vi "Main.vi"(10 "DAQ Type":enum16{"Hardware", "Simulation"}(ring), 11 "Module Admin":refnum<class "Delacor_lib_QMH_Module Admin.lvclass">) -> ()   [LabVIEW 2021, in "Func Generator.lvlib"]
doc: "This template is based off of the Queued Message Handler design pattern and the Queued Message Handler project template that ships with LabVIEW.\n\nThe main difference is that the queue is private to this module and communication between modules is performed via Broadcast and Request events.\n\nRequest events are wrapped in public API methods and are handled in the Event Handling Loop (EHL) of this VI. Any module can register for Broadcast events sent by this module. The EHL generates messages based on user interface actions.\n\nThe Message Handling Loop (MHL) processes messages generated by the EHL, or by other messages. The messages are string values, so new messages can be added easily to the Message Cases case structure in the MHL. Each message cluster can also provide an optional value for Message Data, which is a variant that can be converted to whatever message-specific data is required.\n_____\nBased on DQMH Project Template 6.1.0.94."
uses:
  Func Generator.lvlib
  <vilib>/Delacor/Delacor QMH/Libraries/Module Admin_class/Delacor_lib_QMH_Module Admin.lvclass
  Class/Agilent 33210A/Agilent 33210A.lvclass
  C:/repository/common_ATE/Libraries/Func Generator/Class/Abstract/Abstract.lvclass
  Class/Abstract/Abstract.lvclass
  Module Data--cluster.ctl
  Instrument Setting.ctl
  <vilib>/Delacor/Delacor QMH/Libraries/Message Queue_class/Delacor_lib_QMH_Message Queue.lvclass/Delacor_lib_QMH_Message Queue.ctl
  Stop Argument--cluster.ctl
  <vilib>/Delacor/Delacor QMH/Libraries/Module Admin_class/Delacor_lib_QMH_Module Admin.lvclass/Delacor_lib_QMH_Module Admin.ctl
  REQ Initialize Hardware Argument--cluster.ctl
  REQ Initialize Hardware (Reply Payload)--cluster.ctl
  REQ Enable Output Argument--cluster.ctl
  REQ Set Output Impedance Argument--cluster.ctl
  REQ Config Std Waveform Argument--cluster.ctl
  REQ Config Freq Sweep Argument--cluster.ctl
  REQ Self Test Argument--cluster.ctl
  REQ Close Ref Argument--cluster.ctl
  <vilib>/Utility/miscctls.llb/LVPointTypeDef.ctl
  <vilib>/Delacor/Delacor QMH/Libraries/Message Queue_class/Delacor_lib_QMH_Enqueue Message (Single).vi
  <vilib>/Delacor/Delacor QMH/Libraries/Module Admin_class/Delacor_lib_QMH_Get External Launch.vi
  <vilib>/Utility/error.llb/Error Cluster From Error Code.vi
  <vilib>/ErrorRing/Error Ring.xnode
  <vilib>/Delacor/Delacor QMH/Libraries/Message Queue_class/Delacor_lib_QMH_Message Queue.lvclass
panel:
  out "error out":errorcluster
  out "Status":string
  in  "Simulate MHL Error":bool
  in  "Simulate EHL Error":bool
  # "Other QMH Modules communicate with this Module via its Public API (wrappers for its Request Events).\n\nThis Module communicates with other Modules via its Broadcast Events.\nAny module that wants to get these messages, just registers for this module's Broadcast events."
  # "This template is for the Delacor Modified Queued Message Handler design pattern.\n\nSee the block diagram for more information on how to use this template."
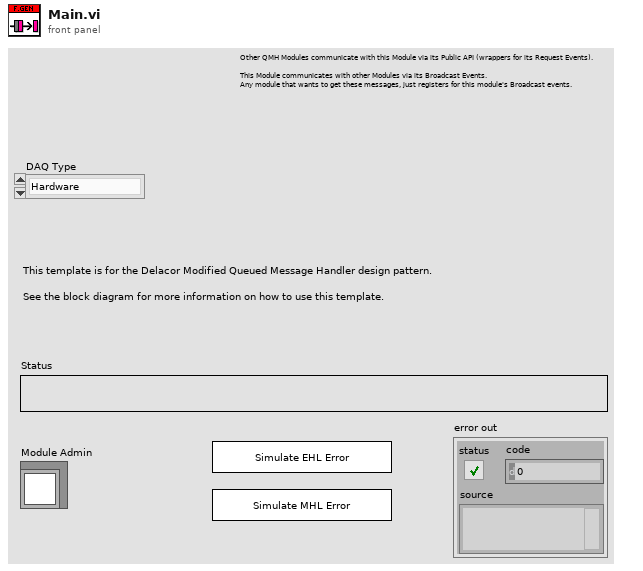
[diagram p1: front panel]
types:
  T1 = typedef "Func Generator.lvlib/Request Events--cluster.ctl" = cluster{"Stop Module":refnum<user-event>, "Show Panel":refnum<user-event>, "Hide Panel":refnum<user-event>, "Get Module Execution Status":refnum<user-event>, "Show Diagram":refnum<user-event>, "REQ Initialize Hardware":refnum<user-event>, "REQ Enable Output":refnum<user-event>, "REQ Set Output Impedance":refnum<user-event>, "REQ Config Std Waveform":refnum<user-event>, "REQ Config Freq Sweep":refnum<user-event>, "REQ Self Test":refnum<user-event>, "REQ Close Ref":refnum<user-event>}
  T2 = typedef "Func Generator.lvlib/Module Data--cluster.ctl" = cluster{"Status":string, "Abstract.lvclass":refnum<class "Abstract.lvclass">, "Connection Setting":T3}
  T3 = typedef "Func Generator.lvlib/Instrument Setting.ctl" = cluster{"Connection Ref":variant, "Serial Configuration":cluster{"Baud Rate":u32, "Parity":u16, "Data Bits":u16, "Flow Control":u16}}
  T4 = enum32{"invalid lock state", "Not Locked", "Locked (No Password)", "Password-protected"}
  T5 = typedef "Func Generator.lvlib/Stop Argument--cluster.ctl" = cluster{"Origin":string, "Exit via Stop Module Req?":bool, "Wait for Module to stop?":bool}
  T6 = typedef "Func Generator.lvlib/REQ Initialize Hardware Argument--cluster.ctl" = cluster{"Connection Setting":T3, "Wait Notifier":refnum<notifier>, "wait for reply":bool}
  T7 = typedef "Func Generator.lvlib/REQ Enable Output Argument--cluster.ctl" = cluster{"Output":bool}
  T8 = typedef "Func Generator.lvlib/REQ Set Output Impedance Argument--cluster.ctl" = cluster{"User-Defined Impedance (50 Ohms)":dbl, "Impedance (0: 50 Ohms)":u16}
  T9 = typedef "Func Generator.lvlib/REQ Config Std Waveform Argument--cluster.ctl" = cluster{"Std Waveform Setting":cluster{"Waveform Function (1: Sine)":u16, "Frequency (1000 Hz)":dbl, "Amplitude (1)":dbl, "Unit (0: Vpp)":u16, "DC Offset (0.00 V)":dbl}}
  T10 = typedef "Func Generator.lvlib/REQ Config Freq Sweep Argument--cluster.ctl" = cluster{"Freq Sweep Setting":cluster{"Sweep Spacing (0: Linear)":u16, "Sweep Time (1.00 s)":dbl, "Stop  Frequency (1000.0 Hz)":dbl, "Start Frequency (100.0 Hz)":dbl, "Enable/Disable Freq Sweep":bool}}
  T11 = typedef "Func Generator.lvlib/REQ Self Test Argument--cluster.ctl" = cluster{"Boolean":bool}
  T12 = typedef "Func Generator.lvlib/REQ Close Ref Argument--cluster.ctl" = cluster{"Boolean":bool}
  T13 = typedef "LVPointTypeDef.ctl" = cluster{"Horizontal":i16, "Vertical":i16}
  T14 = enum32{"Invalid", "Standard", "Closed", "Hidden", "Minimized", "Maximized"}
  T15 = typedef "Func Generator.lvlib/REQ Initialize Hardware (Reply Payload)--cluster.ctl" = cluster{"Connect?":bool, "error":errorcluster}
  T16 = cluster{"Waveform Function (1: Sine)":u16, "Frequency (1000 Hz)":dbl, "Amplitude (1)":dbl, "Unit (0: Vpp)":u16, "DC Offset (0.00 V)":dbl}
  T17 = cluster{"Sweep Spacing (0: Linear)":u16, "Sweep Time (1.00 s)":dbl, "Stop  Frequency (1000.0 Hz)":dbl, "Start Frequency (100.0 Hz)":dbl, "Enable/Disable Freq Sweep":bool}
  T18 = typedef "Instrument Setting.ctl" = cluster{"Connection Ref":variant, "Serial Configuration":cluster{"Baud Rate":u32, "Parity":u16, "Data Bits":u16, "Flow Control":u16}}
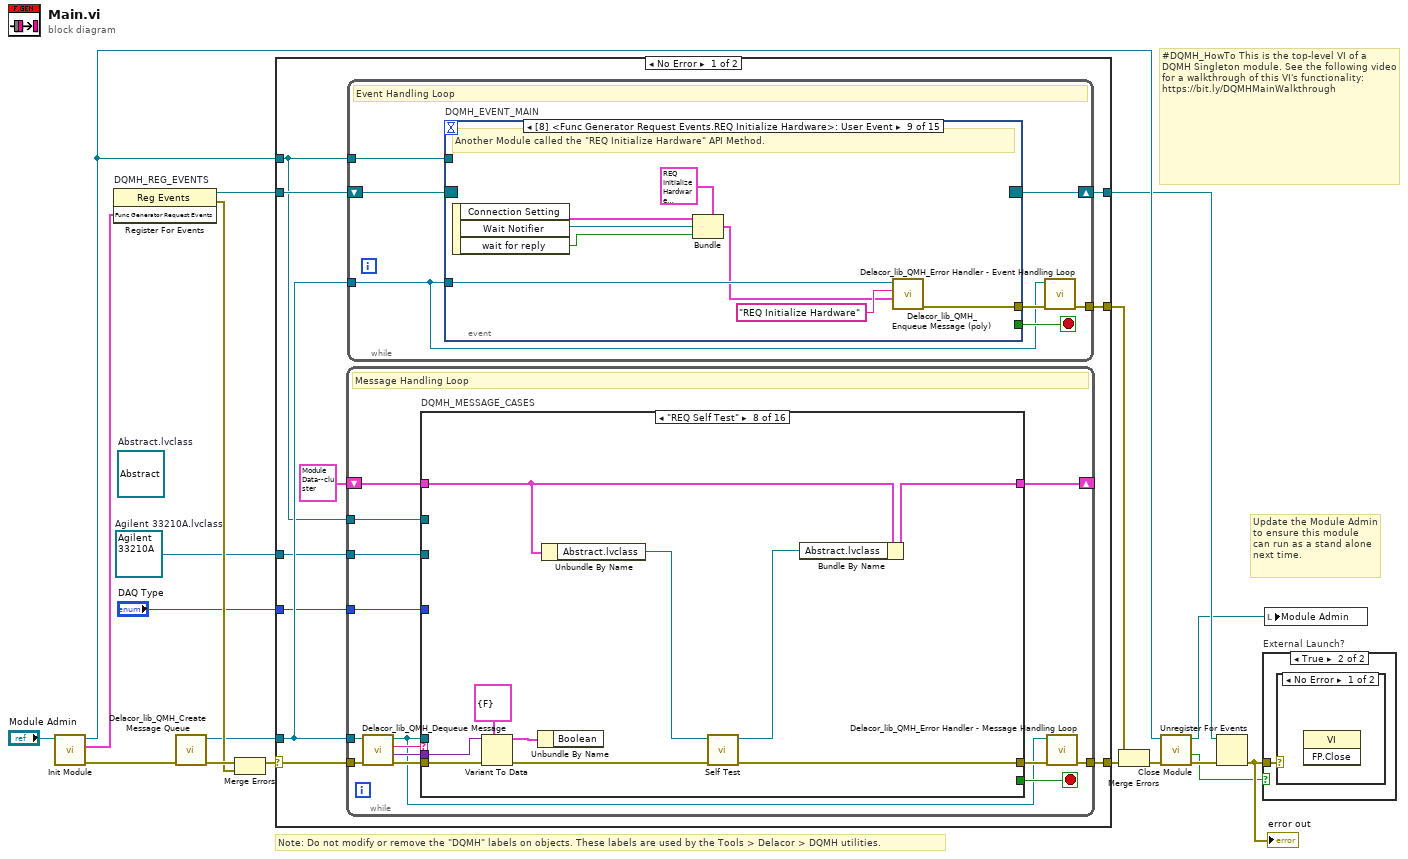
[diagram p0: block diagram]
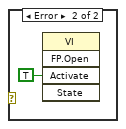
[diagram p3: hidden frame]
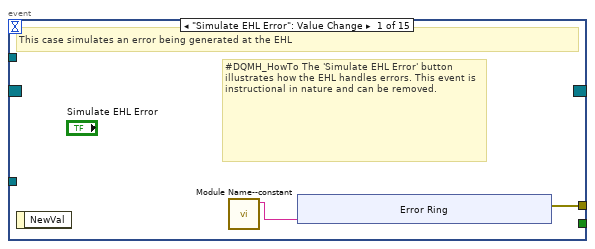
[diagram p4: hidden frame]
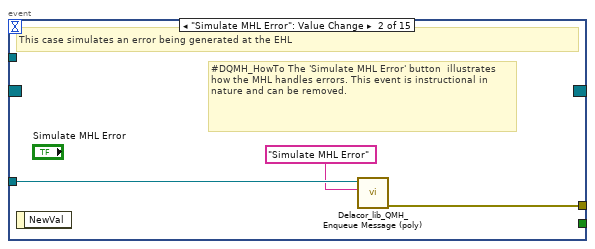
[diagram p5: hidden frame]
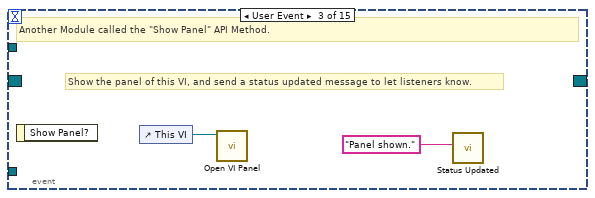
[diagram p6: hidden frame]
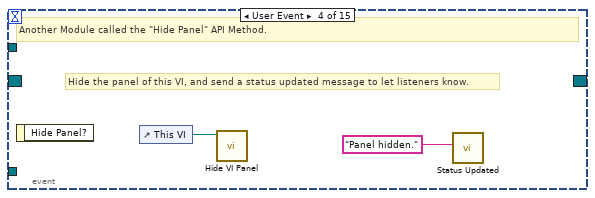
[diagram p7: hidden frame]
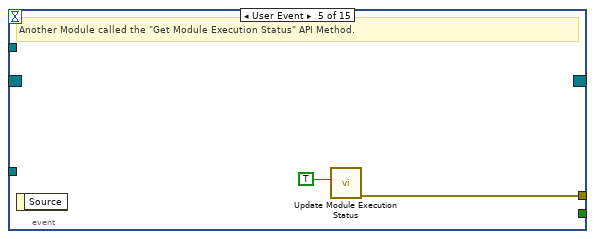
[diagram p8: hidden frame]
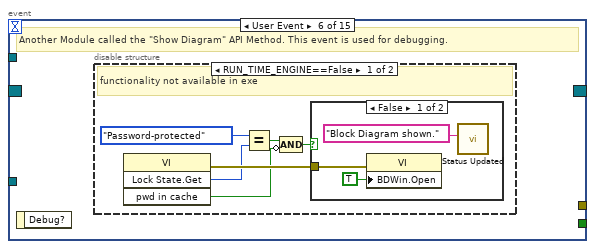
[diagram p9: hidden frame]
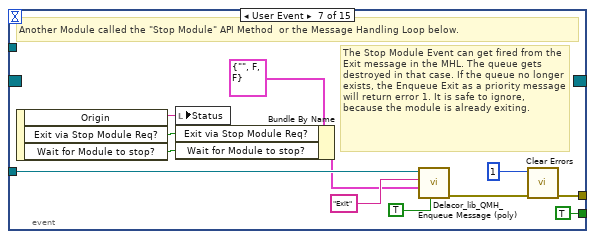
[diagram p12: hidden frame]
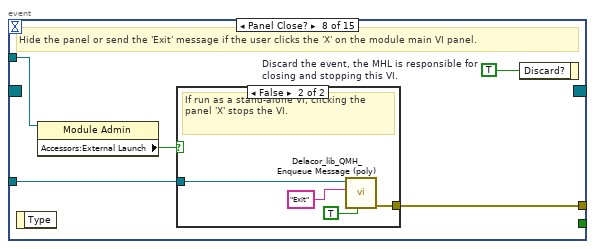
[diagram p13: hidden frame]
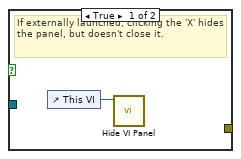
[diagram p14: hidden frame]
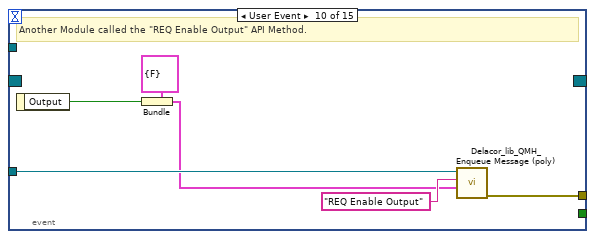
[diagram p15: hidden frame]
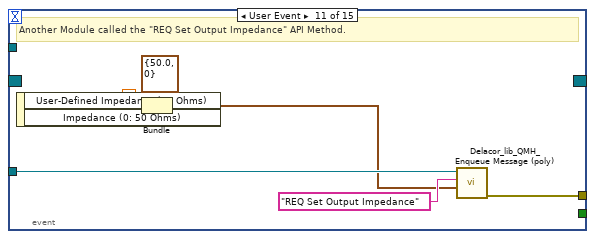
[diagram p16: hidden frame]
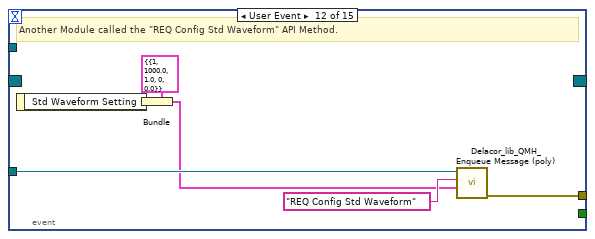
[diagram p17: hidden frame]
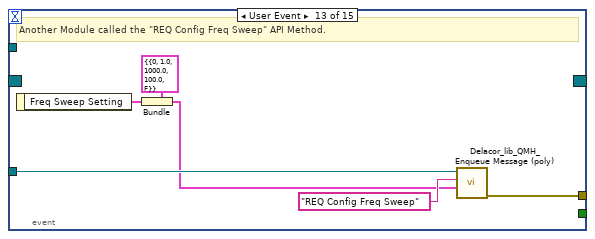
[diagram p18: hidden frame]
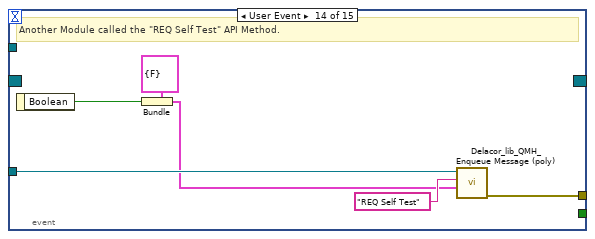
[diagram p19: hidden frame]
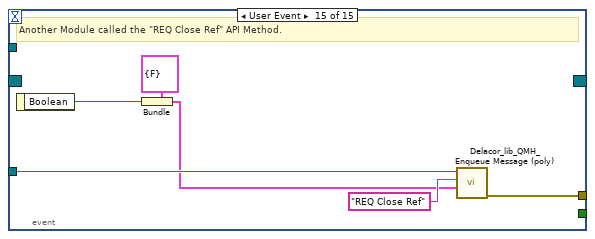
[diagram p20: hidden frame]
diagram:
  w2 = refnum<class "Agilent 33210A.lvclass"> refnum  # Agilent 33210A.lvclass
  (unwired) refnum<class "Abstract.lvclass"> refnum  # Abstract.lvclass
  # "#DQMH_HowTo This is the top-level VI of a DQMH Singleton module. See the following video for a walkthrough of this VI's functionality: https://bit.ly/DQMHMainWalkthrough"
  # "Note: Do not modify or remove the \"DQMH\" labels on objects. These labels are used by the Tools > Delacor > DQMH utilities."
  # "Update the Module Admin to ensure this module can run as a stand alone next time."
  n1 = call "Init Module.vi"("Singleton Module Admin in"="Module Admin") -> ("error out"=w18:errorcluster, "Func Generator Request Events"=w7:T1, "Singleton Module Admin out"=w10:refnum<class "Delacor_lib_QMH_Module Admin.lvclass">)  [unwired: 8 in]
  n2 = register-events "DQMH_REG_EVENTS"(w7) -> (reference out=w8:refnum<event-registration>, error out=w11:errorcluster)  [unwired: 2 in]
  n3 = call <vilib>:"Delacor_lib_QMH_Create Message Queue.vi"("error in"=w18) -> ("error out"=w13:errorcluster, "Message Queue"=w6:refnum<class "Delacor_lib_QMH_Message Queue.lvclass">)  [unwired: 9 in]
  n4 = Merge Errors(w13, w11) -> (w12:errorcluster)
  n5 = case shown="No Error" w12 {
    selector: w12 -> [w27 w331]
    tunnel: [w29 w330] -> w19
    tunnel: [w26 w336] -> w9
    tunnel: w8 -> [w24 w336]
    tunnel: w6 -> [w23 w329]
    tunnel: [w28 _] -> w16
    tunnel: w10 -> [w22 w332]
    tunnel: w2 -> [w21 _]
    tunnel: "DAQ Type" -> [w20 _]
    frame No Error {
      n6 = while {
        tunnel: w23 -> [w135]
        shift-right: [w139] -> _
        shift-left: T2 {"Status"="", "Abstract.lvclass"=refnum, "Connection Setting"={"Connection Ref"=variant, "Serial Configuration"={"Baud Rate"=9600, "Parity"=0, "Data Bits"=8, "Flow Control"=4}}} ("Data Cluster") -> [w140]
        tunnel: w27 -> [w143]
        tunnel: [w141] -> w29
        tunnel: w22 -> [w133]
        tunnel: w21 -> [w132]
        tunnel: w20 -> [w131]
        stop <- w138 stop-if-true
        # "Message Handling Loop"
        n7 = call-dynamic "Delacor_lib_QMH_Dequeue Message.vi"("error in"=w143, "Message Queue in"=w135) -> ("error out"=w142:errorcluster, "Message Data"=w136:variant, "Message"=w137:string, "Message Queue out"=w134:refnum<class "Delacor_lib_QMH_Message Queue.lvclass">)  [unwired: 6 in]
        n8 = case "DQMH_MESSAGE_CASES" shown="\"REQ Self Test\"" w137 {
          selector: w137 -> [_ _ _ _ _ _ _ _ _ _ _ _ _ _ _ w316]
          tunnel: w134 -> [_ _ _ _ _ _ _ _ w248 _ _ _ _ w281 w309 _]
          tunnel: w142 -> [w163 w167 w185 w198 w210 w221 w232 w242 w250 w261 w264 w266 w271 w288 w314 w318]
          tunnel: [w161 w167 w173 w188 w199 w212 w222 w233 w249 w252 w263 w266 w270 w284 w311 w319] -> w144
          tunnel: w140 -> [w152 w166 w169 w192 w205 w216 w226 w237 w246 w256 w262 w265 w268 w283 w299 w317]
          tunnel: [w151 w166 w175 w190 w201 w214 w224 w235 w246 w254 w262 w265 w268 w283 w297 w317] -> w139
          tunnel: [_ _ _ _ _ _ _ _ _ _ _ _ _ _ w308 _] -> w138
          tunnel: w136 -> [_ _ w184 w197 w209 w220 w231 w241 _ w260 _ _ _ w282 w307 _]
          tunnel: w133 -> [w153 _ _ _ _ _ _ _ _ _ _ _ _ w280 w302 _]
          tunnel: w132 -> [w145 _ _ _ _ _ _ _ _ _ _ _ _ _ _ _]
          tunnel: w131 -> [_ _ w176 _ _ _ _ _ _ _ _ _ _ _ _ _]
          frame "Initialize" {
            w147 = "Initial Message" ("Initial Message")
            # "Initialize - Any operation that needs to be done before the module can receive messages. Synchronize Caller Events.vi will inform Start Module.vi that the module has launched and is ready to receive messages. Module Did Init.vi will broadcast that the module initialized."
            n9 = call "Synchronize Caller Events.vi"("error in (no error)"=w163, "Singleton Module Admin in"=w153) -> ("error out"=w162:errorcluster, "Singleton Module Admin out"=w148:refnum<class "Delacor_lib_QMH_Module Admin.lvclass">)  [unwired: 8 in]
            n10 = property class="Module Admin"(reference=w148) -> ("Accessors:External Launch"=w157:bool)  [unwired: 1 in, 2 out]
            n11 = Select(t=T14."Hidden" ("State"), s=w157, f=T14."Standard" ("State")) -> (s? t:f=w154:T14)
            n12 = call "Module Name--constant.vi"() -> ("Module Name"=w160:string)  [unwired: 11 in]
            n13 = property class="VI"("Front Panel.Title"=w160) -> (reference out=w159:refnum<vi>, error out=w165:errorcluster)  [unwired: 2 in]
            n14 = call "Module Name--constant.vi"() -> ("Module Name"=w149:string)  [unwired: 11 in]
            n15 = Bundle By Name(cluster=w152, "Status"=w147, "Abstract.lvclass"=w145) -> (w151:T2)
            n16 = invoke class="VI" method="FP.Open"(reference=w159, error in=w165, "State"=w154) -> (reference out=w158:refnum<vi>, error out=w164:errorcluster)  [unwired: 2 in, 3 out]
            n17 = call "Module Did Init.vi"("error in (no error)"=w162, "Initialized?"=TRUE, "Origin"=w149) -> ("error out"=w161:errorcluster)  [unwired: 8 in]
            n18 = invoke class="VI" method="FP.Center"(reference=w158, error in=w164) -> ()  [unwired: 1 in, 3 out]
            n19 = property on="Pane" class="Pane"("Origin"=T13 {"Horizontal"=0, "Vertical"=0}) -> ()  [unwired: 2 in, 2 out]
            "Status" <- w147
          }
          frame "---Module Specific---" {
            # "Separator -- The following cases handle messages specific to this Module."
          }
          frame "REQ Initialize Hardware" {
            n20 = Variant To Data(error in=w185, type=T6 {"Connection Setting"={"Connection Ref"=variant, "Serial Configuration"={"Baud Rate"=9600, "Parity"=0, "Data Bits"=8, "Flow Control"=4}}, "Wait Notifier"=refnum, "wait for reply"=FALSE} ("REQ Initialize Hardware Argument"), Variant=w184) -> (data=w182:T6, error out=w177:errorcluster)
            n21 = Unbundle By Name(w182) -> ("Wait Notifier"=w181:refnum<notifier>, "wait for reply"=w180:bool, "Connection Setting"=w170:T3)
            n22 = Unbundle By Name(w169) -> ("Abstract.lvclass"=w168:refnum<class "Abstract.lvclass">)
            n23 = call-dynamic "Initialize Hardware.vi"("error in (no error)"=w177, "DAQ Type"=w176, "Connection Setting"=w170, "Abstract in"=w168) -> ("error out"=w173:errorcluster, "Abstract out"=w174:refnum<class "Abstract.lvclass">)  [unwired: 6 in]
            n24 = Bundle By Name(cluster=w169, "Connection Setting"=w170, "Abstract.lvclass"=w174) -> (w175:T2)
            n25 = Unbundle By Name(w173) -> ("status"=w172:bool)
            n26 = Not(x=w172) -> (.not. x?=w171:bool)
            n27 = Bundle By Name(cluster=T15 {"Connect?"=FALSE, "error"={"status"=FALSE, "code"=0, "source"=""}} ("REQ Initialize Hardware (Reply Payload)"), "Connect?"=w171) -> (w179:T15)
            n28 = case shown="True" w180 {
              tunnel: w181 -> [_ w187]
              tunnel: w179 -> [_ w186]
              frame False {
              }
              frame True {
                n29 = Send Notification(notification=w186, notifier=w187) -> ()  [unwired: 1 in, 2 out]
              }
            }
          }
          frame "REQ Enable Output" {
            n30 = Variant To Data(error in=w198, type=T7 {"Output"=FALSE} ("REQ Enable Output Argument"), Variant=w197) -> (data=w195:T7, error out=w194:errorcluster)
            n31 = Unbundle By Name(w195) -> ("Output"=w193:bool)
            n32 = Unbundle By Name(w192) -> ("Abstract.lvclass"=w191:refnum<class "Abstract.lvclass">)
            n33 = call-dynamic "Enable Output.vi"("error in (no error)"=w194, "Output"=w193, "Abstract in"=w191) -> ("error out"=w188:errorcluster, "Abstract out"=w189:refnum<class "Abstract.lvclass">)  [unwired: 7 in]
            n34 = Bundle By Name(cluster=w192, "Abstract.lvclass"=w189) -> (w190:T2)
          }
          frame "REQ Set Output Impedance" {
            n35 = Variant To Data(error in=w210, type=T8 {"User-Defined Impedance (50 Ohms)"=50.0, "Impedance (0: 50 Ohms)"=0} ("REQ Set Output Impedance Argument"), Variant=w209) -> (data=w207:T8, error out=w206:errorcluster)
            n36 = Unbundle By Name(w207) -> ("Impedance (0: 50 Ohms)"=w203:u16, "User-Defined Impedance (50 Ohms)"=w202:dbl)
            n37 = Unbundle By Name(w205) -> ("Abstract.lvclass"=w204:refnum<class "Abstract.lvclass">)
            n38 = call-dynamic "Set Output Impedance.vi"("error in (no error)"=w206, "User-Defined Impedance (50 Ohms)"=w202, "Impedance (0: 50 Ohms)"=w203, "Abstract in"=w204) -> ("error out"=w199:errorcluster, "Abstract out"=w200:refnum<class "Abstract.lvclass">)  [unwired: 6 in]
            n39 = Bundle By Name(cluster=w205, "Abstract.lvclass"=w200) -> (w201:T2)
          }
          frame "REQ Config Std Waveform" {
            n40 = Variant To Data(error in=w221, type=T9 {"Std Waveform Setting"={"Waveform Function (1: Sine)"=1, "Frequency (1000 Hz)"=1000.0, "Amplitude (1)"=1.0, "Unit (0: Vpp)"=0, "DC Offset (0.00 V)"=0.0}} ("REQ Config Std Waveform Argument"), Variant=w220) -> (data=w218:T9, error out=w217:errorcluster)
            n41 = Unbundle By Name(w218) -> ("Std Waveform Setting"=w211:T16)
            n42 = Unbundle By Name(w216) -> ("Abstract.lvclass"=w215:refnum<class "Abstract.lvclass">)
            n43 = call-dynamic "Configure Standard Waveform.vi"("error in (no error)"=w217, "Std Waveform Setting"=w211, "Abstract in"=w215) -> ("error out"=w212:errorcluster, "Abstract out"=w213:refnum<class "Abstract.lvclass">)  [unwired: 7 in]
            n44 = Bundle By Name(cluster=w216, "Abstract.lvclass"=w213) -> (w214:T2)
          }
          frame "REQ Config Freq Sweep" {
            n45 = Variant To Data(error in=w232, type=T10 {"Freq Sweep Setting"={"Sweep Spacing (0: Linear)"=0, "Sweep Time (1.00 s)"=1.0, "Stop  Frequency (1000.0 Hz)"=1000.0, "Start Frequency (100.0 Hz)"=100.0, "Enable/Disable Freq Sweep"=FALSE}} ("REQ Config Freq Sweep Argument"), Variant=w231) -> (data=w229:T10, error out=w228:errorcluster)
            n46 = Unbundle By Name(w229) -> ("Freq Sweep Setting"=w227:T17)
            n47 = Unbundle By Name(w226) -> ("Abstract.lvclass"=w225:refnum<class "Abstract.lvclass">)
            n48 = call-dynamic "Configure Frequency Sweep.vi"("error in (no error)"=w228, "Freq Sweep Setting"=w227, "Abstract in"=w225) -> ("error out"=w222:errorcluster, "Abstract out"=w223:refnum<class "Abstract.lvclass">)  [unwired: 7 in]
            n49 = Bundle By Name(cluster=w226, "Abstract.lvclass"=w223) -> (w224:T2)
          }
          frame "REQ Self Test" {
            n50 = Variant To Data(error in=w242, type=T11 {"Boolean"=FALSE} ("REQ Self Test Argument"), Variant=w241) -> (data=w239:T11, error out=w238:errorcluster)
            n51 = Unbundle By Name(w239) -> ()  [unwired: 1 out]
            n52 = Unbundle By Name(w237) -> ("Abstract.lvclass"=w236:refnum<class "Abstract.lvclass">)
            n53 = call-dynamic "Self Test.vi"("error in (no error)"=w238, "Abstract in"=w236) -> ("error out"=w233:errorcluster, "Abstract out"=w234:refnum<class "Abstract.lvclass">)  [unwired: 8 in]
            n54 = Bundle By Name(cluster=w237, "Abstract.lvclass"=w234) -> (w235:T2)
          }
          frame "REQ Reconnect" {
            # "Duplicate this frame when creating new messages.  Change this comment in the duplicated frame to describe this message."
            n55 = Unbundle By Name(w246) -> ("Connection Setting"=w245:T3)
            n56 = Bundle By Name(cluster=T6 {"Connection Setting"={"Connection Ref"=variant, "Serial Configuration"={"Baud Rate"=9600, "Parity"=0, "Data Bits"=8, "Flow Control"=4}}, "Wait Notifier"=refnum, "wait for reply"=FALSE} ("REQ Initialize Hardware Argument"), "Connection Setting"=w245) -> (w244:T6)
            n57 = Wait (ms)(milliseconds to wait=u32 2000) -> ()  [unwired: 1 out]
            n58 = call-poly <vilib>:"Delacor_lib_QMH_Enqueue Message (poly).vi"("error in"=w250, "Message Data"=w244, "Message"="REQ Initialize Hardware", "Message Queue in"=w248) -> ("error out"=w249:errorcluster)  [unwired: 6 in, 1 out]
          }
          frame "REQ Close Ref" {
            n59 = Variant To Data(error in=w261, type=T12 {"Boolean"=FALSE} ("REQ Close Ref Argument"), Variant=w260) -> (data=w258:T12, error out=w257:errorcluster)
            n60 = Unbundle By Name(w258) -> ()  [unwired: 1 out]
            n61 = Unbundle By Name(w256) -> ("Abstract.lvclass"=w255:refnum<class "Abstract.lvclass">)
            n62 = call-dynamic "Close Ref.vi"("error in (no error)"=w257, "Abstract in"=w255) -> ("error out"=w252:errorcluster, "Abstract out"=w253:refnum<class "Abstract.lvclass">)  [unwired: 8 in]
            n63 = Bundle By Name(cluster=w256, "Abstract.lvclass"=w253) -> (w254:T2)
          }
          frame "---Copy This Frame---" {
            # "Duplicate this frame when creating new messages.  Change this comment in the duplicated frame to describe this message."
            n64 = Merge Errors(w264) -> (w263:errorcluster)
          }
          frame "---Exit and Error Handling---" {
            # "Separator - The following cases handle errors and exit messages."
          }
          frame "Simulate MHL Error" {
            # "#DQMH_HowTo The 'Simulate MHL Error' button  illustrates how the MHL handles errors. This event is instructional in nature and can be removed."
            # "Simulate an error occurring at the MHL"
            n65 = call "Module Name--constant.vi"() -> ("Module Name"=w267:string)  [unwired: 11 in]
            n66 = xnode "Error Ring"("parameter 0"=w267) -> ("error out"=w269:errorcluster)
            n67 = Merge Errors(w271, w269) -> (w270:errorcluster)
          }
          frame "Error" {
            # "#CodeRecommended - If you ever change the name of this \"Error\" message, you'll need to update the name in the Check Loop Error.vi as well."
            # "#CodeRecommended - If the module is running in standalone mode (External Launch = FALSE), this code will pop up an error dialog and call the 'Exit' message if an error occurs. Add more fine-grained error handling here."
            # "Error - Check the error message data and respond accordingly. This message is sent by the \"Error Handler\" VIs at the end of each loop in this application."
            n68 = property class="Module Admin"(reference=w280) -> ("Accessors:External Launch"=w279:bool)  [unwired: 1 in, 2 out]
            n69 = Variant To Data(error in=w288, type=errorcluster {"status"=FALSE, "code"=0, "source"=""} ("error constant"), Variant=w282) -> (data=w289:errorcluster, error out=w286:errorcluster)
            n70 = call "Error Reported.vi"("Error"=w289) -> ()  [unwired: 10 in, 1 out]
            n71 = case shown="False" w279 {
              tunnel: [w294 _] -> w285
              tunnel: w281 -> [w292 _]
              tunnel: w289 -> [w293 _]
              frame False {
                n72 = call <vilib>:"Simple Error Handler.vi"("error in (no error)"=w293) -> ()  [unwired: 4 in, 5 out]
                n73 = call-poly <vilib>:"Delacor_lib_QMH_Enqueue Message (poly).vi"("Priority Message? (F)"=TRUE, "Message"="REQ Reconnect ", "Message Queue in"=w292) -> ("error out"=w294:errorcluster)  [unwired: 7 in, 1 out]
              }
              frame True {
                # "If the module was launched externally, calling the Error Reported broadcast VI is the only action performed by the \"Error\" message. The module's caller can then process the error appropriately."
              }
            }
            n74 = Merge Errors(w286, w285) -> (w284:errorcluster)
            n75 = local write "error out"(w284) -> ()
          }
          frame "Exit" {
            w306 = 91  # 91: not all Exit messages will have an argument
            w308 = TRUE  # Stop the VI
            # "Release the message queue reference"
            # "Exit - Exit the application."
            n76 = Variant To Data(error in=w314, type=T5 {"Origin"="", "Exit via Stop Module Req?"=FALSE, "Wait for Module to stop?"=FALSE} ("Stop Argument"), Variant=w307) -> (data=w304:T5, error out=w310:errorcluster)
            n77 = call <vilib>:"Clear Errors.vi"("error in (no error)"=w310, "specific error code to clear (0: all)"=w306) -> ("error out"=w313:errorcluster)  [unwired: 4 in, 1 out]
            n78 = control-ref of="This VI"() -> (w303:refnum<vi>)
            n79 = Unbundle By Name(w299) -> ("Abstract.lvclass"=w298:refnum<class "Abstract.lvclass">)
            n80 = call "Handle Exit.vi"("Stop Argument"=w304, "Admin in"=w302, "VI reference"=w303) -> ("error out"=w301:errorcluster)  [unwired: 7 in, 1 out]
            n81 = call-dynamic "Close Ref.vi"("error in (no error)"=w301, "Abstract in"=w298) -> ("error out"=w300:errorcluster, "Abstract out"=w296:refnum<class "Abstract.lvclass">)  [unwired: 8 in]
            n82 = call-dynamic "Delacor_lib_QMH_Release Message Queue.vi"("error in"=w313, "Message Queue"=w309) -> ("error out"=w312:errorcluster)  [unwired: 9 in]
            n83 = Bundle By Name(cluster=w299, "Abstract.lvclass"=w296) -> (w297:T2)
            n84 = call <vilib>:"Clear Errors.vi"("error in (no error)"=w300) -> ("error out"=w295:errorcluster)  [unwired: 5 in, 1 out]
            n85 = Merge Errors(w312, w295) -> (w311:errorcluster)
          }
          frame Default {
            # "'Default' case only runs if there is a message that isn't defined in any of the other cases.  Output a programming error."
            n86 = call "Module Name--constant.vi"() -> ("Module Name"=w315:string)  [unwired: 11 in]
            n87 = xnode "Error Ring"("parameter 0"=w316, "parameter 1"=w315) -> ("error out"=w320:errorcluster)
            n88 = Merge Errors(w318, w320) -> (w319:errorcluster)
          }
        }
        n89 = call-dynamic "Delacor_lib_QMH_Error Handler - Message Handling Loop.vi"("error in"=w144, "Message Queue in"=w134) -> ("dup error in"=w141:errorcluster)  [unwired: 8 in, 1 out]
      }
      n90 = while {
        tunnel: w23 -> [w30]
        shift-right: [w33] -> w26
        shift-left: w24 -> [w34]
        tunnel: [w35] -> w28
        tunnel: w22 -> [w31]
        stop <- w32 stop-if-true
        # "Event Handling Loop"
        n91 = event "DQMH_EVENT_MAIN" shown="[8] <Func Generator Request Events.REQ Initialize Hardware>: User Event" {
          selector: w34 -> [_ _ _ _ _ _ _ _ _ _ _ _ _ _ _]
          dyn-events: [_ _ _ _ _ _ _ _ _ _ _ _ _ _ _] -> w33
          timeout: _ -> [_ _ _ _ _ _ _ _ _ _ _ _ _ _ _]
          tunnel: [_ _ _ _ _ _ TRUE ("Discard?") _ _ _ _ _ _ _ _] -> w32
          tunnel: w30 -> [_ w47 _ _ _ _ w71 w78 w93 w99 w106 w112 w118 w124 w130]
          tunnel: [w38 w48 _ _ w54 _ w74 w80 w86 w94 w100 w107 w113 w119 w125] -> w36
          tunnel: w31 -> [_ _ _ _ _ _ _ w77 _ _ _ _ _ _ _]
          event "Simulate EHL Error": Value Change {
            # "#DQMH_HowTo The 'Simulate EHL Error' button  illustrates how the EHL handles errors. This event is instructional in nature and can be removed."
            # "This case simulates an error being generated at the EHL"
            n92 = event-data() -> ()  [unwired: 1 in, 1 out]
            n93 = call "Module Name--constant.vi"() -> ("Module Name"=w37:string)  [unwired: 11 in]
            n94 = xnode "Error Ring"("parameter 0"=w37) -> ("error out"=w38:errorcluster)
          }
          event "Simulate MHL Error": Value Change {
            # "#DQMH_HowTo The 'Simulate MHL Error' button  illustrates how the MHL handles errors. This event is instructional in nature and can be removed."
            # "This case simulates an error being generated at the EHL"
            n95 = event-data() -> ()  [unwired: 1 in, 1 out]
            n96 = call-poly <vilib>:"Delacor_lib_QMH_Enqueue Message (poly).vi"("Message"="Simulate MHL Error", "Message Queue in"=w47) -> ("error out"=w48:errorcluster)  [unwired: 8 in, 1 out]
          }
          event User Event {
            # "Show the panel of this VI, and send a status updated message to let listeners know."
            # "Another Module called the \"Show Panel\" API Method."
            n97 = event-data() -> ()  [unwired: 1 in, 1 out]
            n98 = control-ref of="This VI"() -> (w50:refnum<vi>)
            n99 = call "Open VI Panel.vi"("VI"=w50) -> ()  [unwired: 10 in, 1 out]
            n100 = call "Status Updated.vi"("Status"="Panel shown." ("format string")) -> ()  [unwired: 10 in, 1 out]
          }
          event User Event {
            # "Hide the panel of this VI, and send a status updated message to let listeners know."
            # "Another Module called the \"Hide Panel\" API Method."
            n101 = event-data() -> ()  [unwired: 1 in, 1 out]
            n102 = control-ref of="This VI"() -> (w52:refnum<vi>)
            n103 = call "Hide VI Panel.vi"("VI"=w52) -> ()  [unwired: 10 in, 1 out]
            n104 = call "Status Updated.vi"("Status"="Panel hidden." ("format string")) -> ()  [unwired: 10 in, 1 out]
          }
          event User Event {
            # "Another Module called the \"Get Module Execution Status\" API Method."
            n105 = event-data() -> ()  [unwired: 1 in, 1 out]
            n106 = call "Update Module Execution Status.vi"("Running?"=TRUE) -> ("error out"=w54:errorcluster)  [unwired: 10 in]
          }
          event User Event {
            # "Another Module called the \"Show Diagram\" API Method. This event is used for debugging."
            n107 = event-data() -> ()  [unwired: 1 in, 1 out]
            n108 = disable-structure shown="RUN_TIME_ENGINE==False" {
              frame condition #0 (active) {
                # "functionality not available in exe"
                n109 = invoke class="VI" method="Lock State.Get"() -> (error out=w60:errorcluster, "Get Lock State"=w59:T4, "pwd in cache"=w56:bool)  [unwired: 4 in, 1 out]
                n110 = Equal?(x=T4."Password-protected", y=w59) -> (x = y?=w57:bool)
                n111 = Compound Arithmetic op=AND(w57, invert w56) -> (w55:bool)
                n112 = case shown="False" w55 {
                  tunnel: w60 -> [w63 _]
                  frame False {
                    n113 = property class="VI"(error in=w63, "BDWin.Open"=TRUE ("Block Diagram Window:Open")) -> ()  [unwired: 1 in, 2 out]
                    n114 = call "Status Updated.vi"("Status"="Block Diagram shown." ("format string")) -> ()  [unwired: 10 in, 1 out]
                  }
                  frame True {
                    # "Password-protected VI, and the password is not in the cache. Do not show the diagram."
                  }
                }
              }
              frame condition #1 {
              }
            }
          }
          event User Event {
            # "The Stop Module Event can get fired from the Exit message in the MHL. The queue gets destroyed in that case. If the queue no longer exists, the Enqueue Exit as a priority message will return error 1. It is safe to ignore, because the module is already exiting."
            # "Another Module called the \"Stop Module\" API Method  or the Message Handling Loop below."
            n115 = event-data() -> ("Origin"=w70:string, "Exit via Stop Module Req?"=w66:bool, "Wait for Module to stop?"=w65:bool)  [unwired: 1 in]
            n116 = local write "Status"(w70) -> ()
            n117 = Bundle By Name(cluster=T5 {"Origin"="", "Exit via Stop Module Req?"=FALSE, "Wait for Module to stop?"=FALSE} ("Stop Argument"), "Exit via Stop Module Req?"=w66, "Wait for Module to stop?"=w65) -> (w64:T5)
            n118 = call-poly <vilib>:"Delacor_lib_QMH_Enqueue Message (poly).vi"("Priority Message? (F)"=TRUE, "Message Data"=w64, "Message"="Exit", "Message Queue in"=w71) -> ("error out"=w75:errorcluster)  [unwired: 6 in, 1 out]
            n119 = call <vilib>:"Clear Errors.vi"("error in (no error)"=w75, "specific error code to clear (0: all)"=1) -> ("error out"=w74:errorcluster)  [unwired: 4 in, 1 out]
          }
          event Panel Close? {
            w79 = TRUE  # Discard the event, the MHL is responsible for closing and stopping this VI.
            # "Hide the panel or send the 'Exit' message if the user clicks the 'X' on the module main VI panel."
            n120 = event-data() -> ()  [unwired: 1 in, 1 out]
            n121 = property class="Module Admin"(reference=w77) -> ("Accessors:External Launch"=w76:bool)  [unwired: 1 in, 2 out]
            n122 = case shown="False" w76 {
              tunnel: w78 -> [_ w84]
              tunnel: [_ w85] -> w80
              frame True {
                # "If externally launched, clicking the 'X' hides the panel, but doesn't close it."
                n123 = control-ref of="This VI"() -> (w81:refnum<vi>)
                n124 = call "Hide VI Panel.vi"("VI"=w81) -> ()  [unwired: 10 in, 1 out]
              }
              frame False {
                # "If run as a stand-alone VI, clicking the panel 'X' stops the VI."
                n125 = call-poly <vilib>:"Delacor_lib_QMH_Enqueue Message (poly).vi"("Priority Message? (F)"=TRUE, "Message"="Exit", "Message Queue in"=w84) -> ("error out"=w85:errorcluster)  [unwired: 7 in, 1 out]
              }
            }
            n126 = event-data("Discard?"=w79) -> ()  [unwired: 1 in, 1 out]
          }
          event User Event {
            # "Another Module called the \"REQ Initialize Hardware\" API Method."
            n127 = event-data() -> ("Connection Setting"=w89:T18, "Wait Notifier"=w88:refnum<notifier>, "wait for reply"=w87:bool)  [unwired: 1 in]
            n128 = Bundle(cluster=T6 {"Connection Setting"={"Connection Ref"=variant, "Serial Configuration"={"Baud Rate"=9600, "Parity"=0, "Data Bits"=8, "Flow Control"=4}}, "Wait Notifier"=refnum, "wait for reply"=FALSE} ("REQ Initialize Hardware Argument"), "Connection Setting"=w89, "Wait Notifier"=w88, "wait for reply"=w87) -> (w90:T6)
            n129 = call-poly <vilib>:"Delacor_lib_QMH_Enqueue Message (poly).vi"("Message Data"=w90, "Message"="REQ Initialize Hardware", "Message Queue in"=w93) -> ("error out"=w86:errorcluster)  [unwired: 7 in, 1 out]
          }
          event User Event {
            # "Another Module called the \"REQ Enable Output\" API Method."
            n130 = event-data() -> ("Output"=w95:bool)  [unwired: 1 in]
            n131 = Bundle(cluster=T7 {"Output"=FALSE} ("REQ Enable Output Argument"), "Output"=w95) -> (w96:T7)
            n132 = call-poly <vilib>:"Delacor_lib_QMH_Enqueue Message (poly).vi"("Message Data"=w96, "Message"="REQ Enable Output", "Message Queue in"=w99) -> ("error out"=w94:errorcluster)  [unwired: 7 in, 1 out]
          }
          event User Event {
            # "Another Module called the \"REQ Set Output Impedance\" API Method."
            n133 = event-data() -> ("User-Defined Impedance (50 Ohms)"=w102:dbl, "Impedance (0: 50 Ohms)"=w101:u16)  [unwired: 1 in]
            n134 = Bundle(cluster=T8 {"User-Defined Impedance (50 Ohms)"=50.0, "Impedance (0: 50 Ohms)"=0} ("REQ Set Output Impedance Argument"), "User-Defined Impedance (50 Ohms)"=w102, "Impedance (0: 50 Ohms)"=w101) -> (w103:T8)
            n135 = call-poly <vilib>:"Delacor_lib_QMH_Enqueue Message (poly).vi"("Message Data"=w103, "Message"="REQ Set Output Impedance", "Message Queue in"=w106) -> ("error out"=w100:errorcluster)  [unwired: 7 in, 1 out]
          }
          event User Event {
            # "Another Module called the \"REQ Config Std Waveform\" API Method."
            n136 = event-data() -> ("Std Waveform Setting"=w108:T16)  [unwired: 1 in]
            n137 = Bundle(cluster=T9 {"Std Waveform Setting"={"Waveform Function (1: Sine)"=1, "Frequency (1000 Hz)"=1000.0, "Amplitude (1)"=1.0, "Unit (0: Vpp)"=0, "DC Offset (0.00 V)"=0.0}} ("REQ Config Std Waveform Argument"), "Std Waveform Setting"=w108) -> (w109:T9)
            n138 = call-poly <vilib>:"Delacor_lib_QMH_Enqueue Message (poly).vi"("Message Data"=w109, "Message"="REQ Config Std Waveform", "Message Queue in"=w112) -> ("error out"=w107:errorcluster)  [unwired: 7 in, 1 out]
          }
          event User Event {
            # "Another Module called the \"REQ Config Freq Sweep\" API Method."
            n139 = event-data() -> ("Freq Sweep Setting"=w114:T17)  [unwired: 1 in]
            n140 = Bundle(cluster=T10 {"Freq Sweep Setting"={"Sweep Spacing (0: Linear)"=0, "Sweep Time (1.00 s)"=1.0, "Stop  Frequency (1000.0 Hz)"=1000.0, "Start Frequency (100.0 Hz)"=100.0, "Enable/Disable Freq Sweep"=FALSE}} ("REQ Config Freq Sweep Argument"), "Freq Sweep Setting"=w114) -> (w115:T10)
            n141 = call-poly <vilib>:"Delacor_lib_QMH_Enqueue Message (poly).vi"("Message Data"=w115, "Message"="REQ Config Freq Sweep", "Message Queue in"=w118) -> ("error out"=w113:errorcluster)  [unwired: 7 in, 1 out]
          }
          event User Event {
            # "Another Module called the \"REQ Self Test\" API Method."
            n142 = event-data() -> ("Boolean"=w120:bool)  [unwired: 1 in]
            n143 = Bundle(cluster=T11 {"Boolean"=FALSE} ("REQ Self Test Argument"), "Boolean"=w120) -> (w121:T11)
            n144 = call-poly <vilib>:"Delacor_lib_QMH_Enqueue Message (poly).vi"("Message Data"=w121, "Message"="REQ Self Test", "Message Queue in"=w124) -> ("error out"=w119:errorcluster)  [unwired: 7 in, 1 out]
          }
          event User Event {
            # "Another Module called the \"REQ Close Ref\" API Method."
            n145 = event-data() -> ("Boolean"=w126:bool)  [unwired: 1 in]
            n146 = Bundle(cluster=T12 {"Boolean"=FALSE} ("REQ Close Ref Argument"), "Boolean"=w126) -> (w127:T12)
            n147 = call-poly <vilib>:"Delacor_lib_QMH_Enqueue Message (poly).vi"("Message Data"=w127, "Message"="REQ Close Ref", "Message Queue in"=w130) -> ("error out"=w125:errorcluster)  [unwired: 7 in, 1 out]
          }
        }
        n148 = call-dynamic "Delacor_lib_QMH_Error Handler - Event Handling Loop.vi"("error in"=w36, "Message Queue in"=w30) -> ("dup error in"=w35:errorcluster)  [unwired: 8 in, 1 out]
      }
    }
    frame Error {
      # "Synchronize Caller Events.vi will inform Start Module.vi that the module has launched and will let the code calling Start Module.vi register for broadcasts and would permit the caller receive the broadcast that an error occurred at launch time."
      n149 = call-dynamic "Delacor_lib_QMH_Release Message Queue.vi"("error in"=w331, "Message Queue"=w329) -> ("error out"=w330:errorcluster)  [unwired: 9 in]
      n150 = call "Synchronize Caller Events.vi"("Singleton Module Admin in"=w332) -> ("error out"=w337:errorcluster)  [unwired: 9 in, 1 out]
      n151 = call "Module Name--constant.vi"() -> ("Module Name"=w335:string)  [unwired: 11 in]
      n152 = Format Into String(format string="An error occurred during initialization. %s is no longer running.", w335) -> (resulting string=w333:string)  [unwired: 2 in, 1 out]
      n153 = Merge Errors(w330, w337) -> (w338:errorcluster)
      n154 = call "Error Reported.vi"("Additional Information"=w333, "Error"=w338) -> ()  [unwired: 9 in, 1 out]
    }
  }
  n155 = Merge Errors(w16, w19) -> (w15:errorcluster)
  n156 = call "Close Module.vi"("error in (no error)"=w15, "Module Admin in"=w10) -> ("error out"=w17:errorcluster, "External Launch"=w3:bool, "Module Admin out"=w4:refnum<class "Delacor_lib_QMH_Module Admin.lvclass">)  [unwired: 7 in]
  n157 = Unregister For Events(event registration refnum=w9, error in=w17) -> (error out=w14:errorcluster)
  "error out" <- w14
  n158 = case "External Launch?" shown="True" w3 {
    tunnel: w14 -> [_ w339]
    frame False {
    }
    frame True {
      n159 = case shown="No Error" w339 {
        frame No Error {
          n160 = invoke class="VI" method="FP.Close"() -> ()  [unwired: 3 in, 3 out]
        }
        frame Error {
          n161 = invoke class="VI" method="FP.Open"("Activate"=TRUE ("Activate?")) -> ()  [unwired: 4 in, 5 out]
        }
      }
    }
  }
  n162 = local write "Module Admin"(w4) -> ()
